vi "CSM Essential States.vi"() -> (3 "CSM Essential States":string[](array[string])=["VI Reference", "Error Handler", "Critical Error", "Target Error", "Target Timeout Error", "Async Response", "Response", "Async Message Posted", "Data: Initialize", "Data: Cleanup", "Macro: Initialize", "Macro: Exit", "Initialize Core Data", "Exit"])   [LabVIEW 2017, in "CSM-Helper Utility.lvlib"]
doc: "### CSM Essential States.vi\n\n-- <b>Indicators</b> --\n- <b>CSM Essential States</b>:"
uses:
  CSM-Helper Utility.lvlib
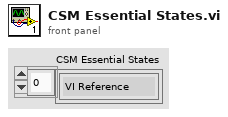
[diagram p1: front panel]
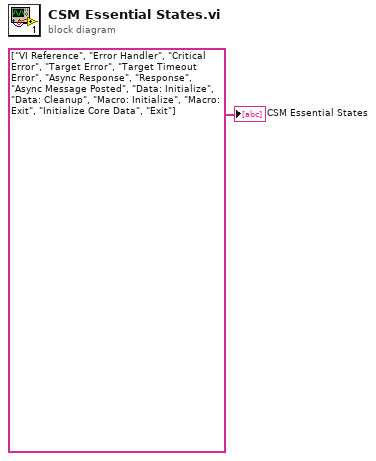
[diagram p0: block diagram]
diagram:
  "CSM Essential States" <- string[] ["VI Reference", "Error Handler", "Critical Error", "Target Error", "Target Timeout Error", "Async Response", "Response", "Async Message Posted", "Data: Initialize", "Data: Cleanup", "Macro: Initialize", "Macro: Exit", "Initialize Core Data", "Exit"] ("Value")
